vi "Main.vi"() -> ()   [LabVIEW 2015, in "Model.lvlib"]
doc: "This template is based off of the Queued Message Handler design pattern and the Queued Message Handler project template that ships with LabVIEW.\n\nThe main difference is that the queue is private to this module and communication between modules is performed via Broadcast and Request events.\n\nRequest events are wrapped in public API methods and are handled in the Event Handling Loop (EHL) of this VI. Any module can register for Broadcast events sent by this module. The EHL generates messages based on user interface actions.\n\nThe Message Handling Loop (MHL) processes messages generated by the EHL, or by other messages. The messages are string values, so new messages can be added easily to the Message Cases case structure in the MHL. Each message cluster can also provide an optional value for Message Data, which is a variant that can be converted to whatever message-specific data is required.\n_____\nBased on Delacor QMH Project Template 4.2.1.64."
uses:
  Model.lvlib
  <vilib>/Delacor/Delacor QMH/Libraries/Module Admin_class/Delacor_lib_QMH_Module Admin.lvclass
  Module Data--cluster.ctl
  <vilib>/Delacor/Delacor QMH/Libraries/Message Queue_class/Delacor_lib_QMH_Message Queue.lvclass/Delacor_lib_QMH_Message Queue.ctl
  Stop Argument--cluster.ctl
  <vilib>/Delacor/Delacor QMH/Libraries/Module Admin_class/Delacor_lib_QMH_Module Admin.lvclass/Delacor_lib_QMH_Module Admin.ctl
  <vilib>/Delacor/Delacor QMH/Libraries/Message Queue_class/Delacor_lib_QMH_Enqueue Message (Single).vi
  <vilib>/Delacor/Delacor QMH/Libraries/Module Admin_class/Delacor_lib_QMH_Get External Launch.vi
  <vilib>/Utility/error.llb/Error Cluster From Error Code.vi
  <vilib>/ErrorRing/Error Ring.xnode
  <vilib>/Delacor/Delacor QMH/Libraries/Message Queue_class/Delacor_lib_QMH_Message Queue.lvclass
  Stock/Stock.lvlib
  Display/Display.lvlib
  Keypad/Keypad.lvlib
  Money/Money.lvlib
panel:
  in  "Simulate MHL Error":bool
  in  "Simulate EHL Error":bool
  in  "Module Admin":refnum<class "Delacor_lib_QMH_Module Admin.lvclass">
  out "Status":string
  out "error out":errorcluster
  # "Message Handler\n\"Model\""
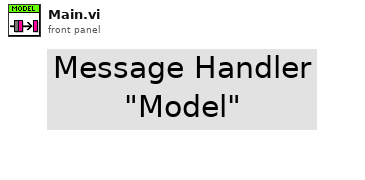
[diagram p1: front panel]
types:
  T1 = typedef "Model.lvlib/Request Events--cluster.ctl" = cluster{"Stop Module":refnum<user-event>, "Show Panel":refnum<user-event>, "Hide Panel":refnum<user-event>, "Get Module Execution Status":refnum<user-event>, "Show Diagram":refnum<user-event>}
  T2 = typedef "Stock.lvlib/Broadcast Events--cluster.ctl" = cluster{"Module Did Init":refnum<user-event>, "Status Updated":refnum<user-event>, "Error Reported":refnum<user-event>, "Module Did Stop":refnum<user-event>, "Update Module Execution Status":refnum<user-event>}
  T3 = typedef "Display.lvlib/Broadcast Events--cluster.ctl" = cluster{"Module Did Init":refnum<user-event>, "Status Updated":refnum<user-event>, "Error Reported":refnum<user-event>, "Module Did Stop":refnum<user-event>, "Update Module Execution Status":refnum<user-event>}
  T4 = typedef "Keypad.lvlib/Broadcast Events--cluster.ctl" = cluster{"Module Did Init":refnum<user-event>, "Status Updated":refnum<user-event>, "Error Reported":refnum<user-event>, "Module Did Stop":refnum<user-event>, "Update Module Execution Status":refnum<user-event>, "Product Selected":refnum<user-event>, "Cancel Request":refnum<user-event>}
  T5 = typedef "Money.lvlib/Broadcast Events--cluster.ctl" = cluster{"Module Did Init":refnum<user-event>, "Status Updated":refnum<user-event>, "Error Reported":refnum<user-event>, "Module Did Stop":refnum<user-event>, "Update Module Execution Status":refnum<user-event>, "Money Entered":refnum<user-event>, "Money Refunded":refnum<user-event>}
  T6 = typedef "Model.lvlib/Module Data--cluster.ctl" = cluster{"Status":string}
  T7 = enum32{"invalid lock state", "Not Locked", "Locked (No Password)", "Password-protected"}
  T8 = typedef "Model.lvlib/Stop Argument--cluster.ctl" = cluster{"Origin":string, "Exit via Stop Module Req?":bool, "Wait for Module to stop?":bool}
  T9 = enum32{"Invalid", "Standard", "Closed", "Hidden", "Minimized", "Maximized"}
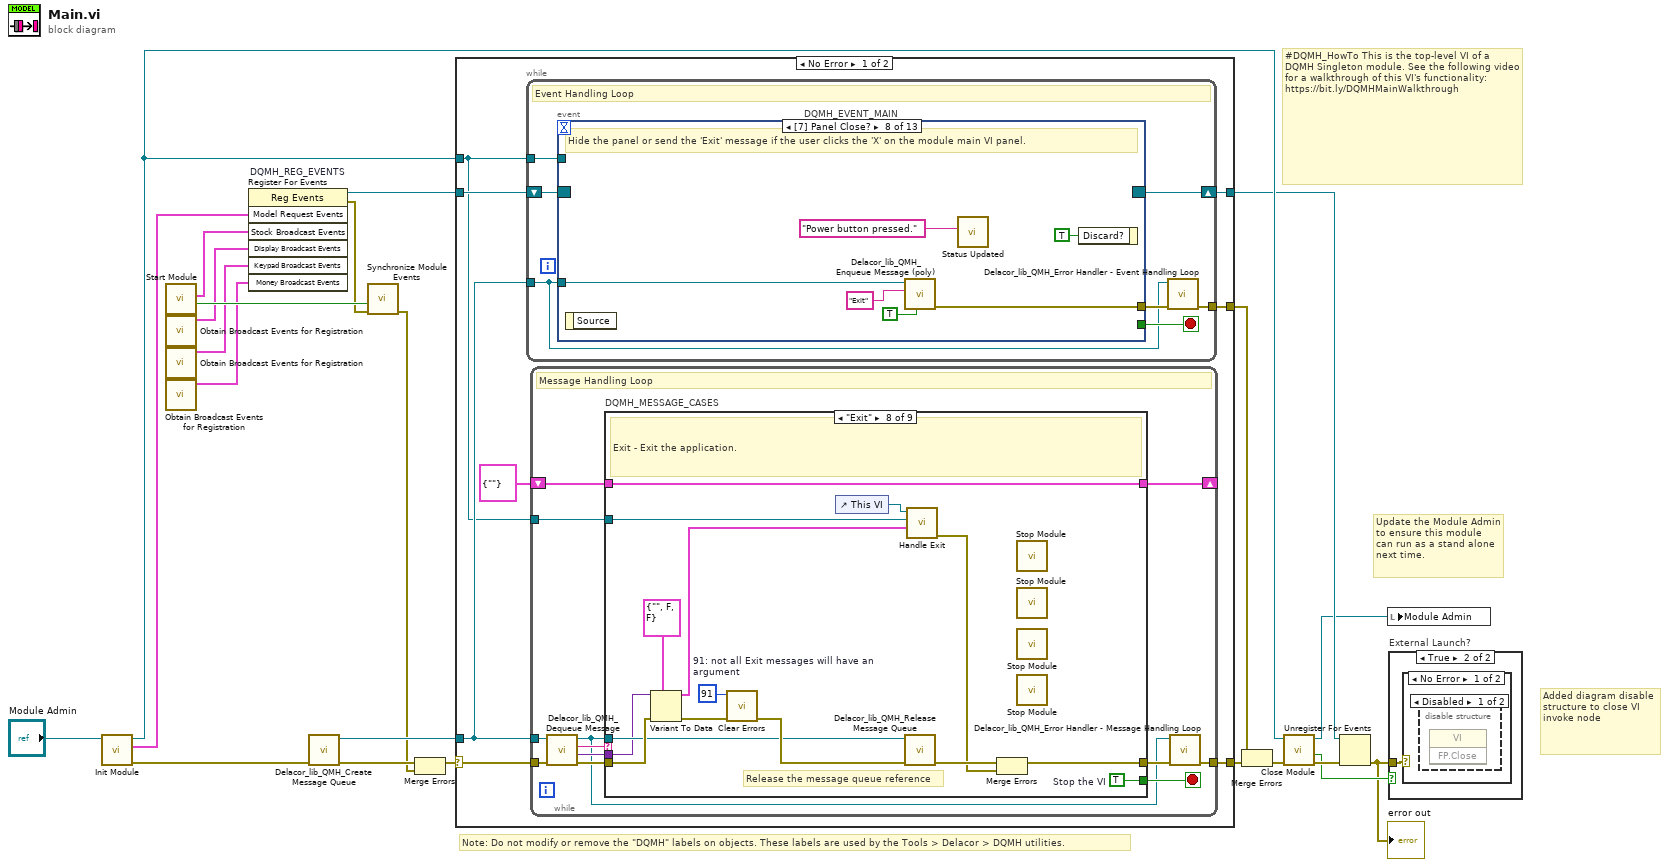
[diagram p0: block diagram]
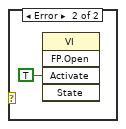
[diagram p4: hidden frame]
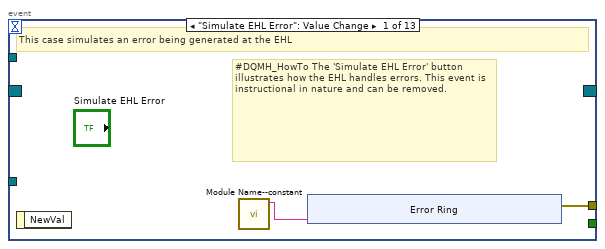
[diagram p5: hidden frame]
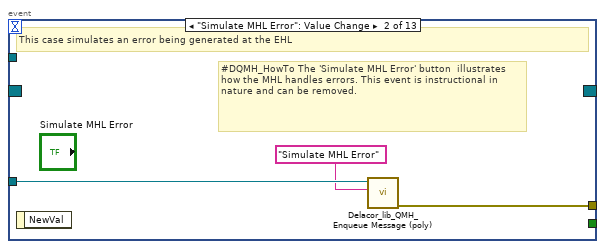
[diagram p6: hidden frame]
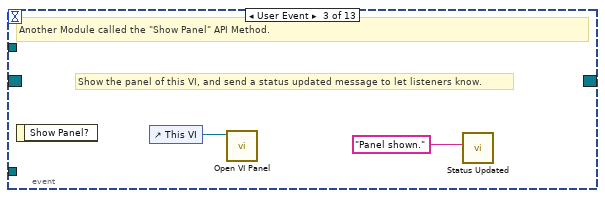
[diagram p7: hidden frame]
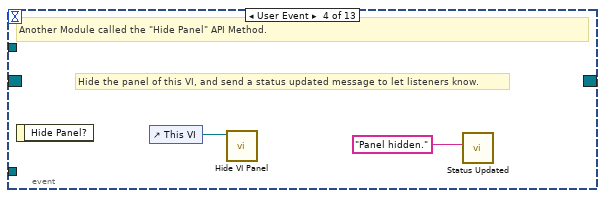
[diagram p8: hidden frame]
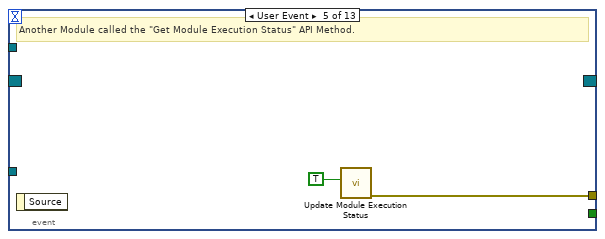
[diagram p9: hidden frame]
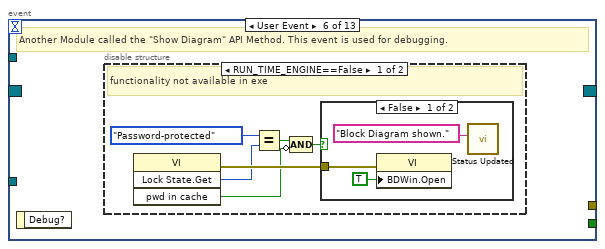
[diagram p10: hidden frame]
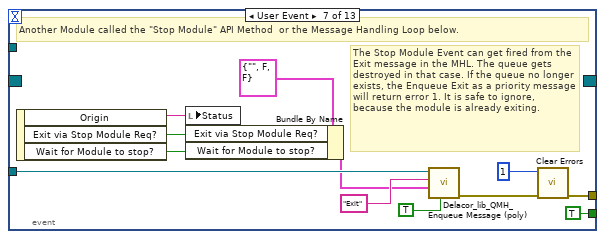
[diagram p13: hidden frame]
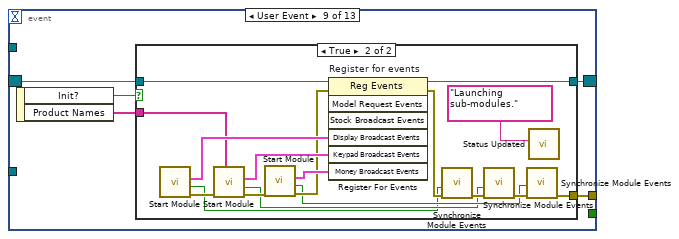
[diagram p14: hidden frame]
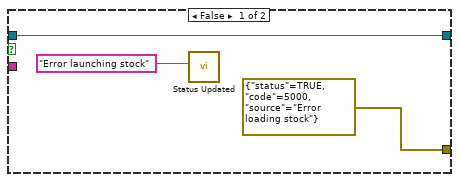
[diagram p15: hidden frame]
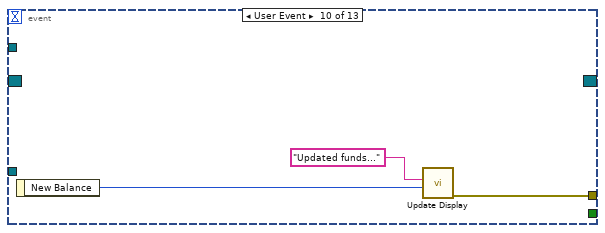
[diagram p16: hidden frame]
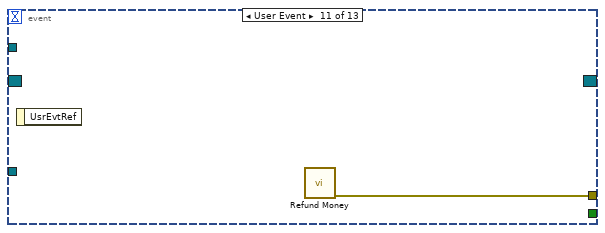
[diagram p17: hidden frame]
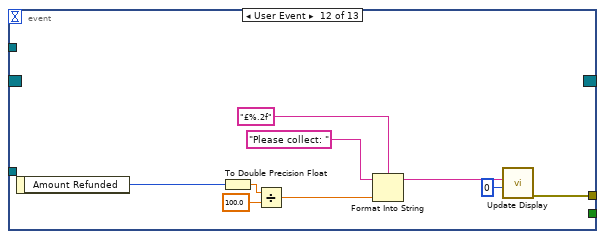
[diagram p18: hidden frame]
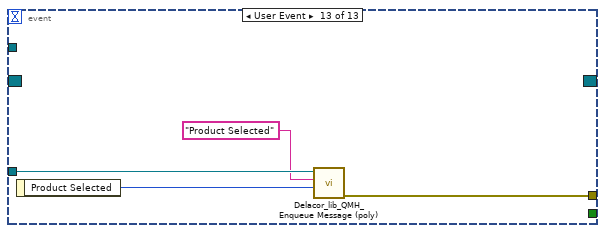
[diagram p19: hidden frame]
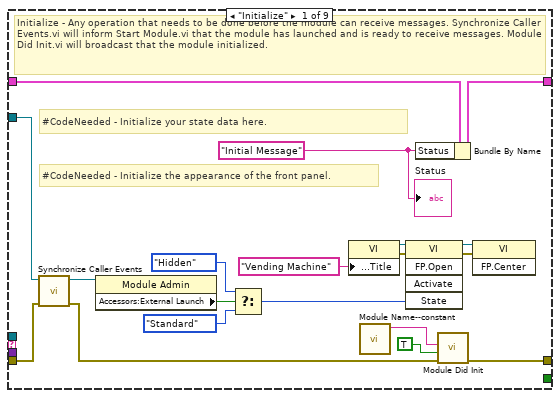
[diagram p20: hidden frame]
diagram:
  # "Added diagram disable structure to close VI invoke node"
  # "#DQMH_HowTo This is the top-level VI of a DQMH Singleton module. See the following video for a walkthrough of this VI's functionality: https://bit.ly/DQMHMainWalkthrough"
  # "Note: Do not modify or remove the \"DQMH\" labels on objects. These labels are used by the Tools > Delacor > DQMH utilities."
  # "Update the Module Admin to ensure this module can run as a stand alone next time."
  n1 = call "Init Module.vi"("Singleton Module Admin in"="Module Admin") -> ("error out"=w22:errorcluster, "Model Request Events"=w13:T1, "Singleton Module Admin out"=w16:refnum<class "Delacor_lib_QMH_Module Admin.lvclass">)  [unwired: 8 in]
  n2 = call "Start Module.vi"() -> ("Wait for Event Sync?"=w8:bool, "Stock Broadcast Events"=w9:T2)  [unwired: 8 in, 2 out]
  n3 = call "Obtain Broadcast Events for Registration.vi"() -> ("Display Broadcast Events"=w5:T3)  [unwired: 9 in, 2 out]
  n4 = call "Obtain Broadcast Events for Registration.vi"() -> ("Keypad Broadcast Events"=w4:T4)  [unwired: 9 in, 2 out]
  n5 = call "Obtain Broadcast Events for Registration.vi"() -> ("Money Broadcast Events"=w3:T5)  [unwired: 9 in, 2 out]
  n6 = register-events "DQMH_REG_EVENTS"(w13, w9, w5, w4, w3) -> (reference out=w14:refnum<event-registration>, error out=w7:errorcluster)  [unwired: 2 in]
  n7 = call <vilib>:"Delacor_lib_QMH_Create Message Queue.vi"("error in (no error)"=w22) -> ("error out"=w18:errorcluster, "Message Queue"=w12:refnum<class "Delacor_lib_QMH_Message Queue.lvclass">)  [unwired: 9 in]
  n8 = call "Synchronize Module Events.vi"("error in (no error)"=w7, "Wait for Event Sync?"=w8) -> ("error out"=w6:errorcluster)  [unwired: 9 in]
  n9 = Merge Errors(w18, w6) -> (w17:errorcluster)
  n10 = case shown="No Error" w17 {
    selector: w17 -> [w29 w231]
    tunnel: [w31 w231] -> w23
    tunnel: [w28 w228] -> w15
    tunnel: w14 -> [w26 w228]
    tunnel: w12 -> [w25 _]
    tunnel: [w30 _] -> w20
    tunnel: w16 -> [w24 w224]
    frame No Error {
      n11 = while {
        tunnel: w25 -> [w32]
        shift-right: [w35] -> w28
        shift-left: w26 -> [w36]
        tunnel: [w37] -> w30
        tunnel: w24 -> [w33]
        stop <- w34 stop-if-true
        # "Event Handling Loop"
        n12 = event "DQMH_EVENT_MAIN" shown="[7] Panel Close?" {
          selector: w36 -> [_ _ _ _ _ _ _ _ w85 _ _ _ _]
          dyn-events: [_ _ _ _ _ _ _ _ w84 _ _ _ _] -> w35
          timeout: _ -> [_ _ _ _ _ _ _ _ _ _ _ _ _]
          tunnel: [_ _ _ _ _ _ TRUE ("Discard?") _ _ _ _ _ _] -> w34
          tunnel: w32 -> [_ w49 _ _ _ _ w73 w82 _ _ _ _ w125]
          tunnel: [w40 w50 _ _ w56 _ w76 w83 w87 w111 w112 w121 w124] -> w38
          tunnel: w33 -> [_ _ _ _ _ _ _ _ _ _ _ _ _]
          event "Simulate EHL Error": Value Change {
            # "#DQMH_HowTo The 'Simulate EHL Error' button  illustrates how the EHL handles errors. This event is instructional in nature and can be removed."
            # "This case simulates an error being generated at the EHL"
            n13 = event-data() -> ()  [unwired: 1 in, 1 out]
            n14 = call "Module Name--constant.vi"() -> ("Module Name"=w39:string)  [unwired: 11 in]
            n15 = xnode "Error Ring"("parameter 0"=w39) -> ("error out"=w40:errorcluster)
          }
          event "Simulate MHL Error": Value Change {
            # "#DQMH_HowTo The 'Simulate MHL Error' button  illustrates how the MHL handles errors. This event is instructional in nature and can be removed."
            # "This case simulates an error being generated at the EHL"
            n16 = event-data() -> ()  [unwired: 1 in, 1 out]
            n17 = call-poly <vilib>:"Delacor_lib_QMH_Enqueue Message (poly).vi"("Message"="Simulate MHL Error", "Message Queue in"=w49) -> ("error out"=w50:errorcluster)  [unwired: 8 in, 1 out]
          }
          event User Event {
            # "Show the panel of this VI, and send a status updated message to let listeners know."
            # "Another Module called the \"Show Panel\" API Method."
            n18 = event-data() -> ()  [unwired: 1 in, 1 out]
            n19 = control-ref of="This VI"() -> (w52:refnum<vi>)
            n20 = call "Open VI Panel.vi"("VI"=w52) -> ()  [unwired: 10 in, 1 out]
            n21 = call "Status Updated.vi"("Status"="Panel shown." ("format string")) -> ()  [unwired: 10 in, 1 out]
          }
          event User Event {
            # "Hide the panel of this VI, and send a status updated message to let listeners know."
            # "Another Module called the \"Hide Panel\" API Method."
            n22 = event-data() -> ()  [unwired: 1 in, 1 out]
            n23 = control-ref of="This VI"() -> (w54:refnum<vi>)
            n24 = call "Hide VI Panel.vi"("VI"=w54) -> ()  [unwired: 10 in, 1 out]
            n25 = call "Status Updated.vi"("Status"="Panel hidden." ("format string")) -> ()  [unwired: 10 in, 1 out]
          }
          event User Event {
            # "Another Module called the \"Get Module Execution Status\" API Method."
            n26 = event-data() -> ()  [unwired: 1 in, 1 out]
            n27 = call "Update Module Execution Status.vi"("Running?"=TRUE) -> ("error out"=w56:errorcluster)  [unwired: 10 in]
          }
          event User Event {
            # "Another Module called the \"Show Diagram\" API Method. This event is used for debugging."
            n28 = event-data() -> ()  [unwired: 1 in, 1 out]
            n29 = disable-structure shown="RUN_TIME_ENGINE==False" {
              frame condition #0 (active) {
                # "functionality not available in exe"
                n30 = invoke class="VI" method="Lock State.Get"() -> (error out=w62:errorcluster, "Get Lock State"=w61:T7, "pwd in cache"=w58:bool)  [unwired: 4 in, 1 out]
                n31 = Equal?(x=T7."Password-protected", y=w61) -> (x = y?=w59:bool)
                n32 = Compound Arithmetic op=AND(w59, invert w58) -> (w57:bool)
                n33 = case shown="False" w57 {
                  tunnel: w62 -> [w65 _]
                  frame False {
                    n34 = property class="VI"(error in=w65, "BDWin.Open"=TRUE ("Block Diagram Window:Open")) -> ()  [unwired: 1 in, 2 out]
                    n35 = call "Status Updated.vi"("Status"="Block Diagram shown." ("format string")) -> ()  [unwired: 10 in, 1 out]
                  }
                  frame True {
                    # "Password-protected VI, and the password is not in the cache. Do not show the diagram."
                  }
                }
              }
              frame condition #1 {
              }
            }
          }
          event User Event {
            # "The Stop Module Event can get fired from the Exit message in the MHL. The queue gets destroyed in that case. If the queue no longer exists, the Enqueue Exit as a priority message will return error 1. It is safe to ignore, because the module is already exiting."
            # "Another Module called the \"Stop Module\" API Method  or the Message Handling Loop below."
            n36 = event-data() -> ("Origin"=w72:string, "Exit via Stop Module Req?"=w68:bool, "Wait for Module to stop?"=w67:bool)  [unwired: 1 in]
            n37 = local write "Status"(w72) -> ()
            n38 = Bundle By Name(cluster=T8 {"Origin"="", "Exit via Stop Module Req?"=FALSE, "Wait for Module to stop?"=FALSE} ("Stop Argument"), "Exit via Stop Module Req?"=w68, "Wait for Module to stop?"=w67) -> (w66:T8)
            n39 = call-poly <vilib>:"Delacor_lib_QMH_Enqueue Message (poly).vi"("Priority Message? (F)"=TRUE, "Message Data"=w66, "Message"="Exit", "Message Queue in"=w73) -> ("error out"=w77:errorcluster)  [unwired: 6 in, 1 out]
            n40 = call <vilib>:"Clear Errors.vi"("error in (no error)"=w77, "specific error code to clear (0: all)"=1) -> ("error out"=w76:errorcluster)  [unwired: 4 in, 1 out]
          }
          event Panel Close? {
            # "Hide the panel or send the 'Exit' message if the user clicks the 'X' on the module main VI panel."
            n41 = event-data() -> ()  [unwired: 1 in, 1 out]
            n42 = call-poly <vilib>:"Delacor_lib_QMH_Enqueue Message (poly).vi"("Priority Message? (F)"=TRUE, "Message"="Exit", "Message Queue in"=w82) -> ("error out"=w83:errorcluster)  [unwired: 7 in, 1 out]
            n43 = call "Status Updated.vi"("Status"="Power button pressed." ("format string")) -> ()  [unwired: 10 in, 1 out]
            n44 = event-data("Discard?"=TRUE) -> ()  [unwired: 1 in, 1 out]
          }
          event User Event {
            n45 = event-data() -> ("Init?"=w88:bool, "Product Names"=w86:string[])  [unwired: 1 in]
            n46 = case shown="True" w88 {
              tunnel: [errorcluster {"status"=TRUE, "code"=5000, "source"="Error loading stock"} ("error constant") w97] -> w87
              tunnel: w86 -> [_ w93]
              tunnel: w85 -> [w90 w108]
              tunnel: [w90 w107] -> w84
              frame False {
                n47 = call "Status Updated.vi"("Status"="Error launching stock" ("format string")) -> ()  [unwired: 10 in, 1 out]
              }
              frame True {
                n48 = call "Start Module.vi"() -> ("error out"=w103:errorcluster, "Wait for Event Sync?"=w94:bool, "Display Broadcast Events"=w106:T3)  [unwired: 8 in, 1 out]
                n49 = call "Start Module.vi"("Product Names"=w93, "error in (no error)"=w103) -> ("error out"=w102:errorcluster, "Wait for Event Sync?"=w95:bool, "Keypad Broadcast Events"=w105:T4)  [unwired: 6 in, 1 out]
                n50 = call "Start Module.vi"("error in (no error)"=w102) -> ("error out"=w101:errorcluster, "Wait for Event Sync?"=w96:bool, "Money Broadcast Events"=w104:T5)  [unwired: 7 in, 1 out]
                n51 = register-events "Register for events"(reference=w108, error in=w101, w106, w105, w104) -> (reference out=w107:refnum<event-registration>, error out=w100:errorcluster)  [unwired: 2 in]
                n52 = call "Synchronize Module Events.vi"("error in (no error)"=w100, "Wait for Event Sync?"=w94) -> ("error out"=w99:errorcluster)  [unwired: 9 in]
                n53 = call "Synchronize Module Events.vi"("error in (no error)"=w99, "Wait for Event Sync?"=w95) -> ("error out"=w98:errorcluster)  [unwired: 9 in]
                n54 = call "Synchronize Module Events.vi"("error in (no error)"=w98, "Wait for Event Sync?"=w96) -> ("error out"=w97:errorcluster)  [unwired: 9 in]
                n55 = call "Status Updated.vi"("Status"="Launching sub-modules." ("format string")) -> ()  [unwired: 10 in, 1 out]
              }
            }
          }
          event User Event {
            n56 = event-data() -> ("New Balance"=w110:u32)  [unwired: 1 in]
            n57 = call "Update Display.vi"("Balance"=w110, "Message to display"="Updated funds...") -> ("error out"=w111:errorcluster)  [unwired: 9 in]
          }
          event User Event {
            n58 = event-data() -> ()  [unwired: 1 in, 1 out]
            n59 = call "Refund Money.vi"() -> ("error out"=w112:errorcluster)  [unwired: 11 in]
          }
          event User Event {
            n60 = event-data() -> ("Amount Refunded"=w115:u32)  [unwired: 1 in]
            n61 = To Double Precision Float(number=w115) -> (double precision float=w118:dbl)
            n62 = Divide(x=w118, y=100.0) -> (x/y=w116:dbl)
            n63 = Format Into String(format string="£%.2f", initial string="Please collect: ", w116) -> (resulting string=w114:string)  [unwired: 1 in, 1 out]
            n64 = call "Update Display.vi"("Balance"=u32 0, "Message to display"=w114) -> ("error out"=w121:errorcluster)  [unwired: 9 in]
          }
          event User Event {
            n65 = event-data() -> ("Product Selected"=w122:u32)  [unwired: 1 in]
            n66 = call-poly <vilib>:"Delacor_lib_QMH_Enqueue Message (poly).vi"("Message Data"=w122, "Message"="Product Selected", "Message Queue in"=w125) -> ("error out"=w124:errorcluster)  [unwired: 7 in, 1 out]
          }
        }
        n67 = call-dynamic "Delacor_lib_QMH_Error Handler - Event Handling Loop.vi"("error in (no error)"=w38, "Message Queue in"=w32) -> ("dup error in"=w37:errorcluster)  [unwired: 8 in, 1 out]
      }
      n68 = while {
        tunnel: w25 -> [w128]
        shift-right: [w132] -> _
        shift-left: T6 {"Status"=""} ("Data Cluster") -> [w133]
        tunnel: w29 -> [w136]
        tunnel: [w134] -> w31
        tunnel: w24 -> [w126]
        stop <- w131 stop-if-true
        # "Message Handling Loop"
        n69 = call-dynamic "Delacor_lib_QMH_Dequeue Message.vi"("error in (no error)"=w136, "Message Queue in"=w128) -> ("error out"=w135:errorcluster, "Message Data"=w129:variant, "Message"=w130:string, "Message Queue out"=w127:refnum<class "Delacor_lib_QMH_Message Queue.lvclass">)  [unwired: 6 in]
        n70 = case "DQMH_MESSAGE_CASES" shown="\"Exit\"" w130 {
          selector: w130 -> [_ _ _ _ _ _ _ _ w211]
          tunnel: w127 -> [_ _ _ _ _ _ w186 w203 _]
          tunnel: w135 -> [w154 w158 w161 w166 w170 w175 w193 w209 w213]
          tunnel: [w152 w158 w160 w162 w170 w174 w189 w206 w214] -> w137
          tunnel: w133 -> [w144 w157 w159 w168 w169 w172 w188 w202 w212]
          tunnel: [w143 w157 w159 w168 w169 w172 w188 w202 w212] -> w132
          tunnel: [_ _ _ _ _ _ _ w201 _] -> w131
          tunnel: w129 -> [_ _ _ w167 _ _ w187 w200 _]
          tunnel: w126 -> [w145 _ _ _ _ _ w185 w195 _]
          frame "Initialize" {
            w139 = "Initial Message" ("Initial Message")
            # "#CodeNeeded - Initialize the appearance of the front panel."
            # "#CodeNeeded - Initialize your state data here."
            # "Initialize - Any operation that needs to be done before the module can receive messages. Synchronize Caller Events.vi will inform Start Module.vi that the module has launched and is ready to receive messages. Module Did Init.vi will broadcast that the module initialized."
            n71 = call "Synchronize Caller Events.vi"("error in (no error)"=w154, "Singleton Module Admin in"=w145) -> ("error out"=w153:errorcluster, "Singleton Module Admin out"=w140:refnum<class "Delacor_lib_QMH_Module Admin.lvclass">)  [unwired: 8 in]
            n72 = property class="Module Admin"(reference=w140) -> ("Accessors:External Launch"=w149:bool)  [unwired: 1 in, 2 out]
            n73 = Select(t=T9."Hidden" ("State"), s=w149, f=T9."Standard" ("State")) -> (s? t:f=w146:T9)
            n74 = property class="VI"("Front Panel.Title"="Vending Machine" ("Front Panel Window:Title")) -> (reference out=w151:refnum<vi>, error out=w156:errorcluster)  [unwired: 2 in]
            n75 = call "Module Name--constant.vi"() -> ("Module Name"=w141:string)  [unwired: 11 in]
            n76 = invoke class="VI" method="FP.Open"(reference=w151, error in=w156, "State"=w146) -> (reference out=w150:refnum<vi>, error out=w155:errorcluster)  [unwired: 2 in, 3 out]
            n77 = Bundle By Name(cluster=w144, "Status"=w139) -> (w143:T6)
            n78 = call "Module Did Init.vi"("error in (no error)"=w153, "Initialized?"=TRUE, "Origin"=w141) -> ("error out"=w152:errorcluster)  [unwired: 8 in]
            n79 = invoke class="VI" method="FP.Center"(reference=w150, error in=w155) -> ()  [unwired: 1 in, 3 out]
            "Status" <- w139
          }
          frame "--- Module Specific ---" {
            # "Separator -- The following cases handle messages specific to this Module."
          }
          frame "---Copy This Frame---" {
            # "Duplicate this frame when creating new messages.  Change this comment in the duplicated frame to describe this message."
            n80 = Merge Errors(w161) -> (w160:errorcluster)
          }
          frame "Product Selected" {
            # "All in one VI to reduce the risk of race conditions"
            # "Check Stock Level, Check Balance\nOutputs: Not in stock,  Insufficient Funds, Accepted (Reduce Stock and Balance"
            n81 = Variant To Data(error in=w166, type=u32 0 ("Product Selected"), Variant=w167) -> (data=w164:u32, error out=w163:errorcluster)
            n82 = call "Despence Product.vi"("error in (no error)"=w163, "Stock Item"=w164) -> ("error out"=w162:errorcluster)  [unwired: 9 in]
          }
          frame "--- Exit and Error Handling---" {
            # "Separator - The following cases handle errors and exit messages."
          }
          frame "Simulate MHL Error" {
            # "#DQMH_HowTo The 'Simulate MHL Error' button  illustrates how the MHL handles errors. This event is instructional in nature and can be removed."
            # "Simulate an error occurring at the MHL"
            n83 = call "Module Name--constant.vi"() -> ("Module Name"=w171:string)  [unwired: 11 in]
            n84 = xnode "Error Ring"("parameter 0"=w171) -> ("error out"=w173:errorcluster)
            n85 = Merge Errors(w175, w173) -> (w174:errorcluster)
          }
          frame "Error" {
            # "If the module is running standalone, then pop up an error dialog and call the \"Exit\" message."
            # "#CodeRecommended - If you ever change the name of this \"Error\" message, you'll need to update the name in the Check Loop Error.vi as well."
            # "#CodeRecommended - If the module is running in standalone mode (External Launch = FALSE), this code will pop up an error dialog and call the 'Exit' message if an error occurs. Add more fine-grained error handling here."
            # "Error - Check the error message data and respond accordingly. This message is sent by the \"Error Handler\" VIs at the end of each loop in this application."
            n86 = property class="Module Admin" props=["Accessors:External Launch"](reference=w185) -> ()  [unwired: 1 in, 3 out]
            n87 = Variant To Data(error in=w193, type=errorcluster {"status"=FALSE, "code"=0, "source"=""} ("error constant"), Variant=w187) -> (data=w194:errorcluster, error out=w191:errorcluster)
            n88 = call "Error Reported.vi"("Error"=w194) -> ()  [unwired: 10 in, 1 out]
            n89 = call <vilib>:"Simple Error Handler.vi"("error in (no error)"=w194) -> ()  [unwired: 4 in, 5 out]
            n90 = call-poly <vilib>:"Delacor_lib_QMH_Enqueue Message (poly).vi"("Priority Message? (F)"=TRUE, "Message"="Exit", "Message Queue in"=w186) -> ("error out"=w190:errorcluster)  [unwired: 7 in, 1 out]
            n91 = Merge Errors(w191, w190) -> (w189:errorcluster)
            n92 = local write "error out"(w189) -> ()
          }
          frame "Exit" {
            w199 = 91  # 91: not all Exit messages will have an argument
            w201 = TRUE  # Stop the VI
            # "Release the message queue reference"
            # "Exit - Exit the application."
            n93 = Variant To Data(error in=w209, type=T8 {"Origin"="", "Exit via Stop Module Req?"=FALSE, "Wait for Module to stop?"=FALSE} ("Stop Argument"), Variant=w200) -> (data=w197:T8, error out=w205:errorcluster)
            n94 = call <vilib>:"Clear Errors.vi"("error in (no error)"=w205, "specific error code to clear (0: all)"=w199) -> ("error out"=w208:errorcluster)  [unwired: 4 in, 1 out]
            n95 = control-ref of="This VI"() -> (w196:refnum<vi>)
            n96 = call-dynamic "Delacor_lib_QMH_Release Message Queue.vi"("error in (no error)"=w208, "Message Queue"=w203) -> ("error out"=w207:errorcluster)  [unwired: 9 in]
            n97 = call "Handle Exit.vi"("Stop Argument"=w197, "Admin in"=w195, "VI reference"=w196) -> ("error out"=w204:errorcluster)  [unwired: 7 in, 1 out]
            n98 = Merge Errors(w207, w204) -> (w206:errorcluster)
            n99 = call "Stop Module.vi"() -> ()  [unwired: 11 in, 1 out]
            n100 = call "Stop Module.vi"() -> ()  [unwired: 11 in, 1 out]
            n101 = call "Stop Module.vi"() -> ()  [unwired: 11 in, 1 out]
            n102 = call "Stop Module.vi"() -> ()  [unwired: 11 in, 1 out]
          }
          frame Default {
            # "'Default' case only runs if there is a message that isn't defined in any of the other cases.  Output a programming error."
            n103 = call "Module Name--constant.vi"() -> ("Module Name"=w210:string)  [unwired: 11 in]
            n104 = xnode "Error Ring"("parameter 0"=w211, "parameter 1"=w210) -> ("error out"=w215:errorcluster)
            n105 = Merge Errors(w213, w215) -> (w214:errorcluster)
          }
        }
        n106 = call-dynamic "Delacor_lib_QMH_Error Handler - Message Handling Loop.vi"("error in (no error)"=w137, "Message Queue in"=w127) -> ("dup error in"=w134:errorcluster)  [unwired: 8 in, 1 out]
      }
    }
    frame Error {
      # "Synchronize Caller Events.vi will inform Start Module.vi that the module has launched and will let the code calling Start Module.vi register for broadcasts and would permit the caller receive the broadcast that an error occurred at launch time."
      n107 = call "Synchronize Caller Events.vi"("Singleton Module Admin in"=w224) -> ("error out"=w229:errorcluster)  [unwired: 9 in, 1 out]
      n108 = call "Module Name--constant.vi"() -> ("Module Name"=w227:string)  [unwired: 11 in]
      n109 = Format Into String(format string="An error occurred during initialization. %s is no longer running.", w227) -> (resulting string=w225:string)  [unwired: 2 in, 1 out]
      n110 = Merge Errors(w231, w229) -> (w230:errorcluster)
      n111 = call "Error Reported.vi"("Additional Information"=w225, "Error"=w230) -> ()  [unwired: 9 in, 1 out]
    }
  }
  n112 = Merge Errors(w20, w23) -> (w19:errorcluster)
  n113 = call "Close Module.vi"("error in (no error)"=w19, "Module Admin in"=w16) -> ("error out"=w21:errorcluster, "External Launch"=w2:bool, "Module Admin out"=w10:refnum<class "Delacor_lib_QMH_Module Admin.lvclass">)  [unwired: 7 in]
  n114 = Unregister For Events(event registration refnum=w15, error in=w21) -> (error out=w1:errorcluster)
  "error out" <- w1
  n115 = local write "Module Admin"(w10) -> ()
  n116 = case "External Launch?" shown="True" w2 {
    tunnel: w1 -> [_ w232]
    frame False {
    }
    frame True {
      n117 = case shown="No Error" w232 {
        frame No Error {
          n118 = disable-structure shown="Disabled" {
            frame Disabled {
              n119 = invoke class="VI" method="FP.Close"() -> ()  [unwired: 3 in, 3 out]
            }
            frame Enabled {
            }
          }
        }
        frame Error {
          n120 = invoke class="VI" method="FP.Open"("Activate"=TRUE ("Activate?")) -> ()  [unwired: 4 in, 5 out]
        }
      }
    }
  }
